vi "Get Pin Based Session Information.vi"(8 "error in (no error)":errorcluster, 10 "session information":T1[](array[typedef]), 11 "pin name":string) -> (0 "error out":errorcluster, 3 "pin based session information":T1[](array[typedef]))   [LabVIEW 2020, in "NIDCPowerSourceDCVoltage.lvlib"]
doc: "Gets the session information for the given pin."
uses:
  NIDCPowerSourceDCVoltage.lvlib
  <vilib>/MeasurementLink/MeasurementLink Session Management Client/RPC Messages/ni_measurementlink_sessionmanagement_v1_SessionInformation.ctl
  <vilib>/MeasurementLink/MeasurementLink Session Management Client/RPC Messages/nidevice_grpc_Session.ctl
  <vilib>/MeasurementLink/MeasurementLink Session Management Client/RPC Messages/ni_measurementlink_sessionmanagement_v1_ChannelMapping.ctl
  <vilib>/MeasurementLink/MeasurementLink Session Management Client/MeasurementLink Session Management Client.lvlib
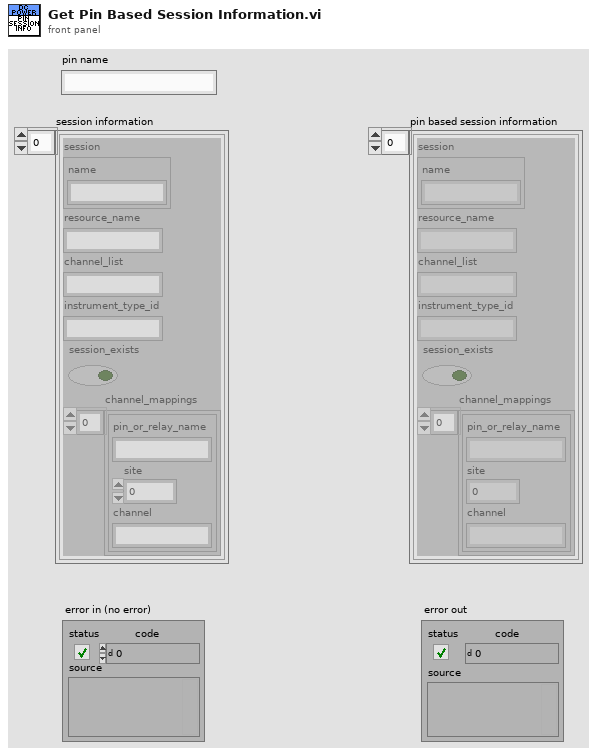
[diagram p1: front panel]
types:
  T1 = typedef "MeasurementLink Session Management Client.lvlib/ni_measurementlink_sessionmanagement_v1_SessionInformation.ctl" = cluster{"session":T2, "resource_name":string, "channel_list":string, "instrument_type_id":string, "session_exists":bool, "channel_mappings":T3[]}
  T2 = typedef "MeasurementLink Session Management Client.lvlib/nidevice_grpc_Session.ctl" = cluster{"name":string}
  T3 = typedef "MeasurementLink Session Management Client.lvlib/ni_measurementlink_sessionmanagement_v1_ChannelMapping.ctl" = cluster{"pin_or_relay_name":string, "site":i32, "channel":string}
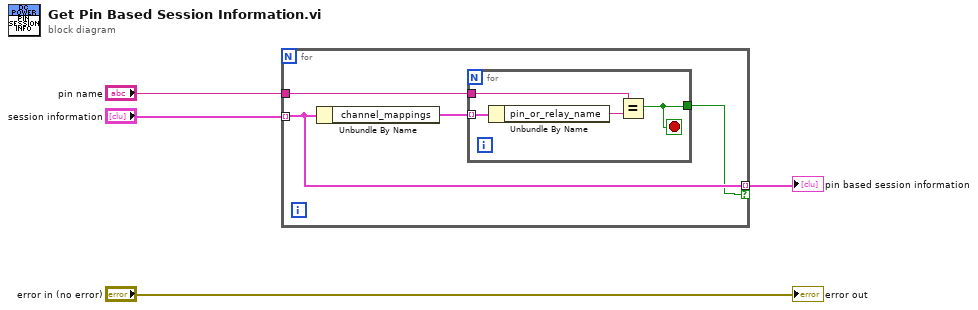
[diagram p0: block diagram]
diagram:
  n1 = for {
    tunnel: "session information" -> [w6] mode=indexing
    tunnel: "pin name" -> [w7]
    tunnel: [w6] -> w2 mode=indexing if=w5
    n2 = Unbundle By Name(w6) -> ("channel_mappings"=w8:T3[])
    n3 = for {
      tunnel: w8 -> [w12] mode=indexing
      tunnel: w7 -> [w10]
      tunnel: [w9] -> w5
      stop <- w9 stop-if-true
      n4 = Unbundle By Name(w12) -> ("pin_or_relay_name"=w11:string)
      n5 = Equal?(x=w10, y=w11) -> (x = y?=w9:bool)
    }
  }
  "pin based session information" <- w2
  "error out" <- "error in (no error)"
